vi "M227 Send Command.vi"(0 "VISA Ref":refnum<visa-resource-name>, 2 "Wait for Reply (T)":bool=TRUE, 7 "Command":string, 11 "Error In":errorcluster) -> (4 "VISA Ref Dup":refnum<visa-resource-name>, 8 "Reply":string, 15 "Error Out":errorcluster)   [LabVIEW 2020]
uses:
  <vilib>/Utility/error.llb/whitespace.ctl
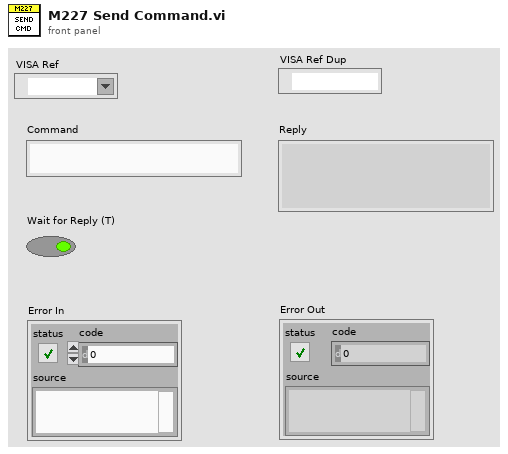
[diagram p1: front panel]
types:
  T1 = typedef "whitespace.ctl" = u16
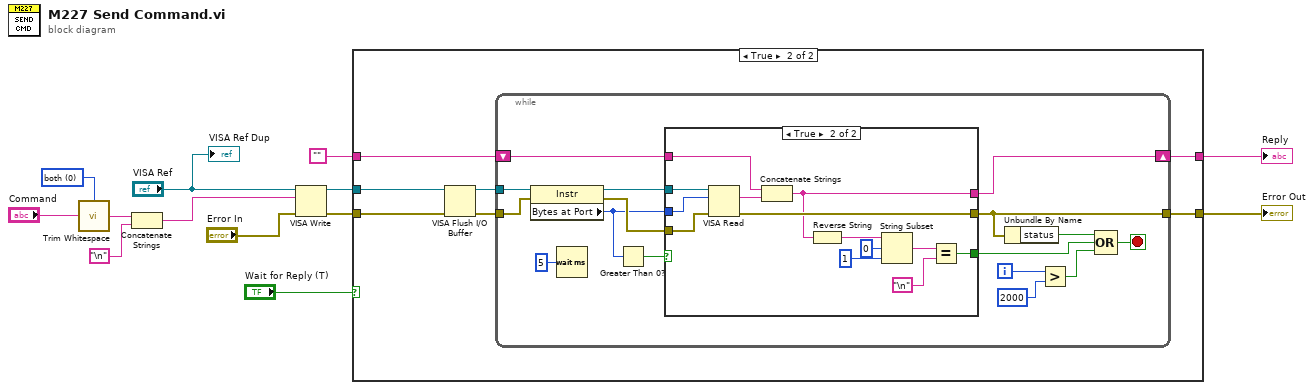
[diagram p0: block diagram]
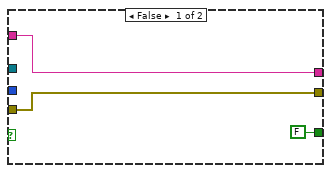
[diagram p3: hidden frame]
diagram:
  w12 = T1 0 items=["both", "start of string", "end of string"] ("location (both)")
  n1 = call <vilib>:"Trim Whitespace.vi"("string"="Command", "location (both)"=w12) -> ("trimmed string"=w11:string)
  n2 = Concatenate Strings(w11, "\n") -> (w9:string)
  n3 = VISA Write(VISA resource name="VISA Ref", write buffer=w9, error in (no error)="Error In") -> (VISA resource name out=w8:refnum<visa-resource-name>, error out=w7:errorcluster)  [unwired: 1 out]
  n4 = case shown="True" "Wait for Reply (T)" {
    tunnel: w8 -> [_ w19]
    tunnel: w7 -> [w15 w17]
    tunnel: "" -> [w14 w22]
    tunnel: [w14 w21] -> w1
    tunnel: [w15 w20] -> w3
    frame False {
    }
    frame True {
      n5 = VISA Flush I/O Buffer(VISA resource name=w19, error in (no error)=w17) -> (VISA resource name out=w18:refnum<visa-resource-name>, error out=w16:errorcluster)  [unwired: 1 in]
      n6 = while {
        tunnel: w18 -> [w38]
        tunnel: w16 -> [w37]
        shift-right: [w26] -> w21
        shift-left: w22 -> [w27]
        tunnel: [w23] -> w20
        i -> [w36]
        stop <- w33 stop-if-true
        n7 = property class="Instr"(reference=w38, error in=w37) -> (reference out=w29:refnum<visa-resource-name>, error out=w30:errorcluster, "Bytes at Port"=w28:u32)
        n8 = Wait (ms)(milliseconds to wait=u32 5) -> ()  [unwired: 1 out]
        n9 = Greater Than 0?(x=w28) -> (x > 0?=w31:bool)
        n10 = case shown="True" w31 {
          tunnel: w30 -> [w40 w53]
          tunnel: w29 -> [_ w54]
          tunnel: w28 -> [_ w52]
          tunnel: w27 -> [w41 w51]
          tunnel: [w41 w48] -> w26
          tunnel: [w40 w49] -> w23
          tunnel: [FALSE w42] -> w24
          frame False {
          }
          frame True {
            n11 = VISA Read(VISA resource name=w54, byte count=w52, error in (no error)=w53) -> (read buffer=w50:string, error out=w49:errorcluster)  [unwired: 2 out]
            n12 = Concatenate Strings(w51, w50) -> (w48:string)
            n13 = Reverse String(1:w48) -> (0:w47:string)
            n14 = String Subset(string=w47, offset (0)=0, length (rest)=1 ("length (rest)")) -> (substring=w44:string)
            n15 = Equal?(x=w44, y="\n") -> (x = y?=w42:bool)
          }
        }
        n16 = Unbundle By Name(w23) -> ("status"=w25:bool)
        n17 = Greater?(x=w36, y=2000) -> (0:w34:bool)
        n18 = Compound Arithmetic op=OR(w25, w24, w34) -> (w33:bool)
      }
    }
  }
  "Reply" <- w1
  "Error Out" <- w3
  "VISA Ref Dup" <- "VISA Ref"
